vi "Parse.vi"(8 "error in (no error)":errorcluster, 10 "Data String":string, 11 "Parser in":refnum<class "Parser.lvclass">) -> (0 "error out":errorcluster, 2 "Data Values":dbl[](array[numeric]), 3 "Parser out":refnum<class "Parser.lvclass">)   [LabVIEW 2018, in "Parser.lvclass"]
doc: "Parserl.lvclass:Parse.vi\n\nThis is the template for the Parse VI for the Parser class.\n\nInstrument Communication Module Version 1.0\nSeptember, 2017 Original Code Consulting David Thomson\n www.originalcode.com"
uses:
  Parser.lvclass
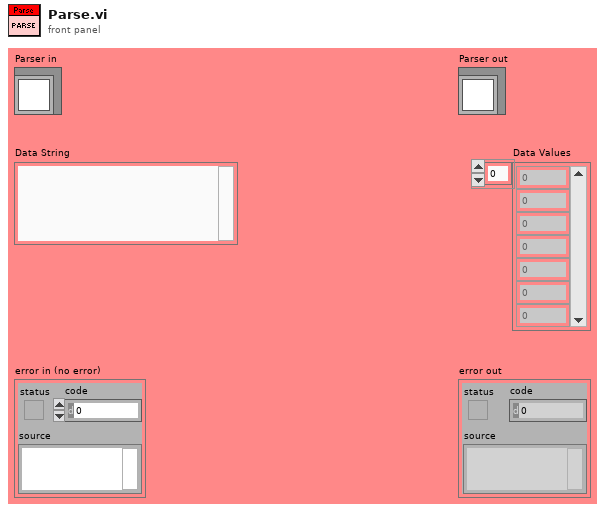
[diagram p1: front panel]
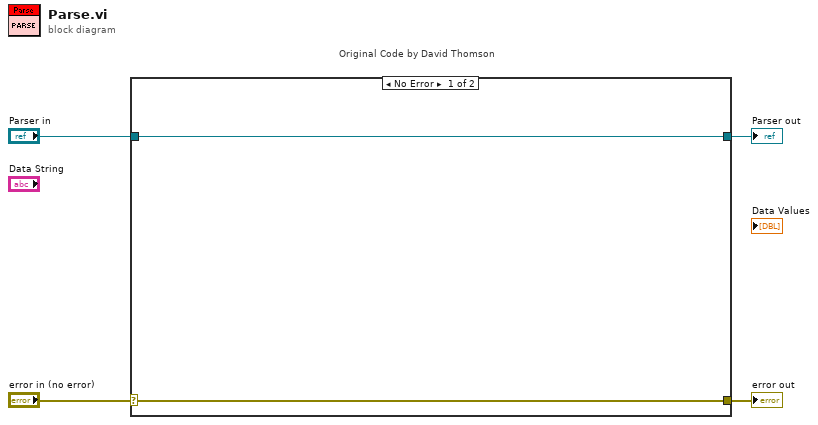
[diagram p0: block diagram]
diagram:
  n1 = case "Original Code by David Thomson" shown="No Error" "error in (no error)" {
    selector: "error in (no error)" -> [w5 w8]
    tunnel: [w5 w8] -> w3
    tunnel: [w6 w7] -> w1
    tunnel: "Parser in" -> [w6 w7]
    frame No Error {
    }
    frame Error {
    }
  }
  "error out" <- w3
  "Parser out" <- w1
